vi "overlay_spots_on_image.vi"(4 "error in":errorcluster, 5 "Selection and Groups":T2[](array[typedef]), 6 "Spots":T3[](array[typedef]) {"Amplitude Correction" step=0.1; "Line Trapping"."Phase Gradient" step=0.05; "Line Trapping"."Vector"."x" step=1e-06 format="%#_6p"; "Line Trapping"."Vector"."y" step=1e-06 format="%#_6p"; "Line Trapping"."Vector"."z" step=1e-06 format="%#_6p"; "NA Position"."r" step=1e-06; "NA Position"."y" step=1e-06; "NA Position"."x" step=1e-06; "Position"."z" step=1e-06; "Position"."y" step=1e-06; "Position"."x" step=1e-06; "Phase" step=0.7753; "Intensity" step=0.1}, 7 "image":T1) -> (0 "error out":errorcluster, 3 "Image":T1(plugin-control))   [LabVIEW 2010]
uses:
  <vilib>/vision/Image Controls.llb/IMAQ Image.ctl
  spot.ctl
  line_trapping.ctl
  selection_element.ctl
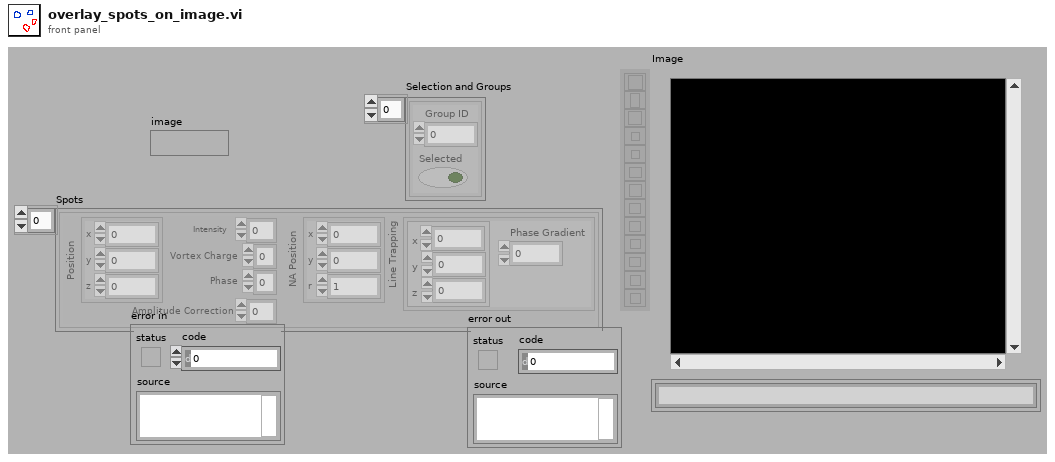
[diagram p1: front panel]
types:
  T1 = typedef "IMAQ Image.ctl" = refnum<image>
  T2 = typedef "selection_element.ctl" = cluster{"Group ID":i32, "Selected":bool}
  T3 = typedef "spot.ctl" = cluster{"Position":cluster{"x":dbl, "y":dbl, "z":dbl}, "Intensity":dbl, "Vortex Charge":i8, "Phase":dbl, "NA Position":cluster{"x":dbl, "y":dbl, "r":dbl}, "Line Trapping":T4, "Amplitude Correction":dbl}
  T4 = typedef "line_trapping.ctl" = cluster{"Vector":cluster{"x":dbl, "y":dbl, "z":dbl}, "Phase Gradient":dbl}
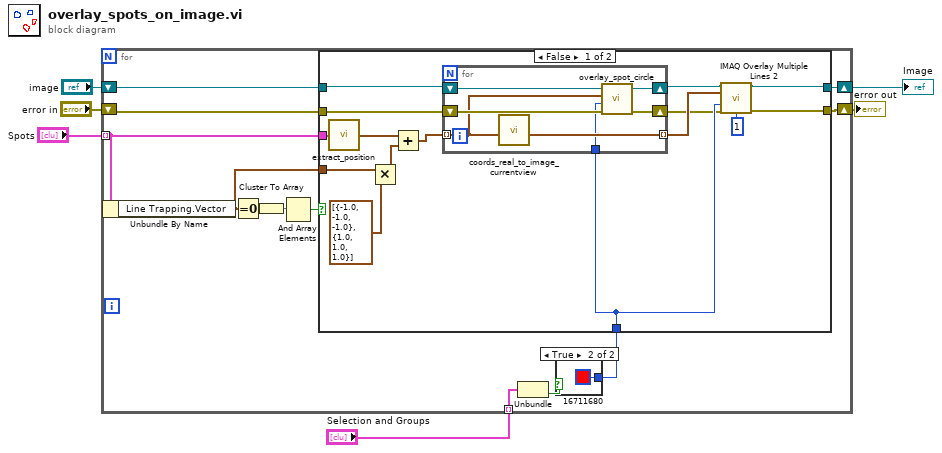
[diagram p0: block diagram]
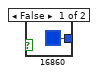
[diagram p2: hidden frame]
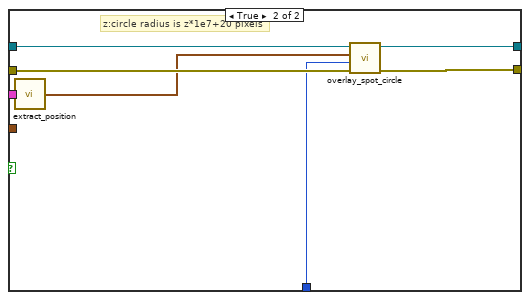
[diagram p3: hidden frame]
diagram:
  n1 = for {
    shift-right: [w17] -> w3
    shift-left: "image" -> [w18]
    tunnel: "Spots" -> [w16] mode=indexing
    tunnel: "Selection and Groups" -> [w12] mode=indexing
    shift-right: [w7] -> w1
    shift-left: "error in" -> [w8]
    n2 = Unbundle By Name(w16) -> ("Line Trapping.Vector"=w10:cluster{"x":dbl, "y":dbl, "z":dbl})
    n3 = Equal To 0?(x=w10) -> (x = 0?=w15:cluster{"x":bool, "y":bool, "z":bool})
    n4 = Cluster To Array(cluster=w15) -> (array=w9:bool[])
    n5 = And Array Elements(Boolean array=w9) -> (logical AND=w14:bool)
    n6 = Unbundle(w12) -> ("Selected"=w13:bool)  [unwired: 1 out]
    n7 = case shown="True" w13 {
      tunnel: [u32 16860 ("color(black)") u32 16711680 ("color(black)")] -> w11
      frame False {
      }
      frame True {
      }
    }
    n8 = case shown="False" w14 {
      tunnel: w18 -> [w31 w48]
      tunnel: [w28 w43] -> w17
      tunnel: w16 -> [w35 w49]
      tunnel: w10 -> [w29 _]
      tunnel: w11 -> [w25 w44]
      tunnel: w8 -> [w22 w47]
      tunnel: [w21 w46] -> w7
      frame False {
        n9 = call "extract_position.vi"("Spot"=w35) -> ("Position"=w33:cluster{"x":dbl, "y":dbl, "z":dbl})
        n10 = Multiply(x=w29, y=cluster{"[0]":dbl, "[1]":dbl, "[2]":dbl}[] [{"[0]"=-1.0, "[1]"=-1.0, "[2]"=-1.0}, {"[0]"=1.0, "[1]"=1.0, "[2]"=1.0}]) -> (x*y=w32:cluster{dbl, dbl, dbl}[])
        n11 = Add(x=w33, y=w32) -> (x+y=w30:cluster{dbl, dbl, dbl}[])
        n12 = for {
          shift-right: [w41] -> w27
          shift-left: w31 -> [w38]
          tunnel: w30 -> [w37] mode=indexing
          tunnel: w25 -> [w36]
          tunnel: [w42] -> w26 mode=indexing
          shift-right: [w40] -> w23
          shift-left: w22 -> [w39]
          n13 = call "coords_real_to_image_currentview.vi"("Position (real coords)"=w37) -> ("Position (pixels, relative to the top left of the image)"=w42:cluster{dbl, dbl})  [unwired: 7 in, 1 out]
          n14 = call "overlay_spot_circle.vi"("error in"=w39, "color(black)"=w36, "Position"=w37, "image"=w38) -> ("error out"=w40:errorcluster, "Image Out"=w41:T1)  [unwired: 3 in]
        }
        n15 = call "IMAQ Overlay Multiple Lines 2"("Image"=w27, "Line End Points"=w26, "Color"=w25, "error in (no error)"=w23, "Width"=u32 1) -> ("Image Out"=w28:T1, "error out"=w21:errorcluster)  [unwired: 9 in]
      }
      frame True {
        # "z:circle radius is z*1e7+20 pixels"
        n16 = call "extract_position.vi"("Spot"=w49) -> ("Position"=w45:cluster{"x":dbl, "y":dbl, "z":dbl})
        n17 = call "overlay_spot_circle.vi"("error in"=w47, "color(black)"=w44, "Position"=w45, "image"=w48) -> ("error out"=w46:errorcluster, "Image Out"=w43:T1)  [unwired: 3 in]
      }
    }
  }
  "Image" <- w3
  "error out" <- w1
